vi "Check Temperature Conversion --Unit Test.vi"() -> ()   [LabVIEW 2021]
uses:
  Controls/Temperature Calibration Array.ctl
  Controls/Temperature Calibration.ctl
panel:
  in  "Expected Temperature Array":dbl[](array[numeric])
  # "200.244, 96.6274, 292.131"
  # "200.244, 96.2528, 274.664"
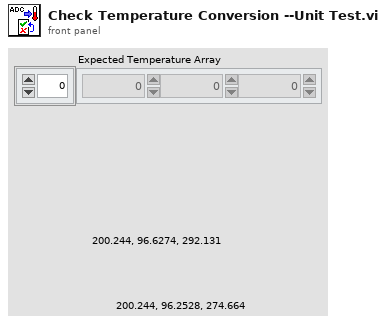
[diagram p1: front panel]
types:
  T1 = typedef "Temperature Calibration Array.ctl" = T2[]
  T2 = typedef "Temperature Calibration.ctl" = cluster{"ADC_to_V_Factor":dbl, "V_to_C_Offset":dbl, "V_to_C_Slope":dbl}
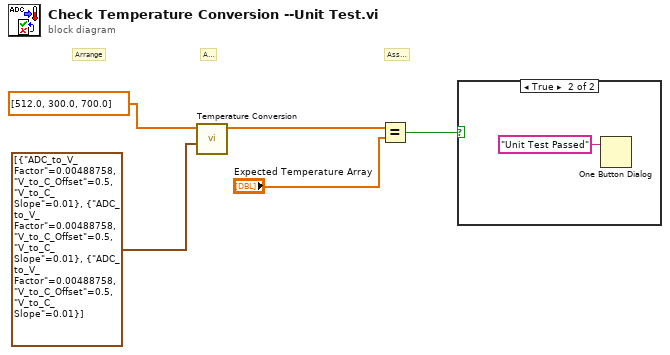
[diagram p0: block diagram]
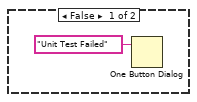
[diagram p2: hidden frame]
diagram:
  # "Assert"
  # "Act"
  # "Arrange"
  n1 = call "Temperature Conversion.vi"("Calibration Array"=T1 [{"ADC_to_V_Factor"=0.00488758, "V_to_C_Offset"=0.5, "V_to_C_Slope"=0.01}, {"ADC_to_V_Factor"=0.00488758, "V_to_C_Offset"=0.5, "V_to_C_Slope"=0.01}, {"ADC_to_V_Factor"=0.00488758, "V_to_C_Offset"=0.5, "V_to_C_Slope"=0.01}], "Raw ADC Array"=dbl[] [512.0, 300.0, 700.0]) -> ("Temperature Array"=w3:dbl[])  [unwired: 9 in]
  n2 = Equal?(x=w3, y="Expected Temperature Array") -> (x = y?=w1:bool)
  n3 = case shown="True" w1 {
    frame False {
      n4 = One Button Dialog(message="Unit Test Failed") -> ()  [unwired: 1 in, 1 out]
    }
    frame True {
      n5 = One Button Dialog(message="Unit Test Passed") -> ()  [unwired: 1 in, 1 out]
    }
  }
